vi "Configure Math.vi"(0 "VISA resource name":refnum<visa-resource-name>, 5 "math function (1:one)":u16(ring)=1 items=["One"=1, "Two"=2], 7 "Enable Math (on:T)":bool=TRUE, 9 "math mode (1:absolute value of deviation)":u16(ring)=1 items=["Absolute Value of Deviation"=1, "Percent of Deviation"=2], 11 "error in (no error)":errorcluster, 12 "reference value (0.0000E+0)":dbl format="%.4e") -> (4 "VISA resource name out":refnum<visa-resource-name>, 15 "error out":errorcluster)   [LabVIEW 2016, in "Agilent 4263X.lvlib"]
doc: "This VI configures the math mode of the instrument."
uses:
  <instrlib>/Agilent 4263X/Agilent 4263X.lvlib
panel:
  # "on\noff"
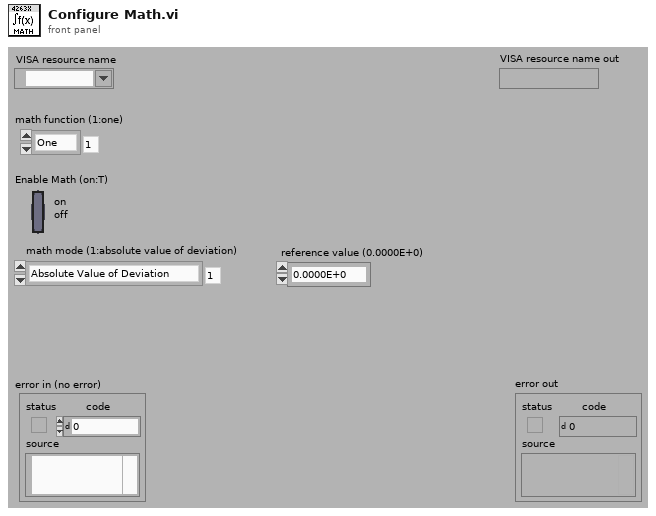
[diagram p1: front panel]
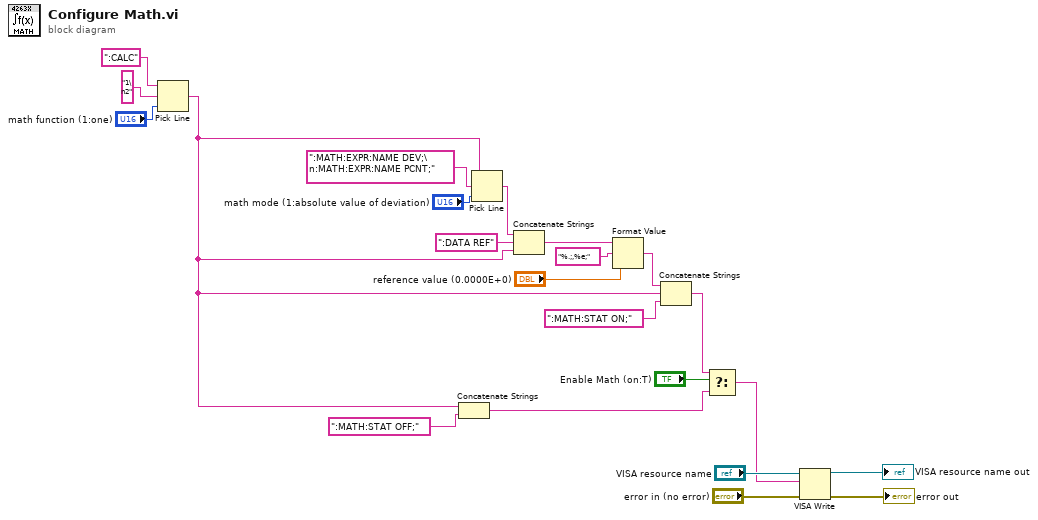
[diagram p0: block diagram]
diagram:
  n1 = Pick Line(string ("")=":CALC", multi-line string="1\n2", line index="math function (1:one)") -> (output string=w2:string)
  n2 = Concatenate Strings(w2, ":MATH:STAT OFF;") -> (w4:string)
  n3 = Pick Line(string ("")=w2, multi-line string=":MATH:EXPR:NAME DEV;\n:MATH:EXPR:NAME PCNT;", line index="math mode (1:absolute value of deviation)") -> (output string=w15:string)
  n4 = Concatenate Strings(w15, ":DATA REF", w2) -> (w13:string)
  n5 = Format Value(string ("")=w13, format string="%.;,%e;", value (0)="reference value (0.0000E+0)") -> (output string=w11:string)
  n6 = Concatenate Strings(w11, w2, ":MATH:STAT ON;") -> (w8:string)
  n7 = Select(t=w8, s="Enable Math (on:T)", f=w4) -> (s? t:f=w7:string)
  n8 = VISA Write(VISA resource name="VISA resource name", write buffer=w7, error in (no error)="error in (no error)") -> (VISA resource name out=→"VISA resource name out":refnum<visa-resource-name>, error out=→"error out":errorcluster)  [unwired: 1 out]
